vi "convertDataNiDAQmx.vi"(8 "error in (no error)":errorcluster, 10 "Data":T1={"Timestamps ms"=[0.0, 0.005, 0.009, 0.012], "Bitmap"=[[TRUE, FALSE, FALSE, FALSE, FALSE, FALSE, FALSE, FALSE, FALSE, TRUE, TRUE, FALSE, FALSE, FALSE, FALSE, FALSE], [FALSE, FALSE, FALSE, FALSE, FALSE, FALSE, FALSE, FALSE, FALSE, FALSE, FALSE, FALSE, FALSE, FALSE, FALSE, TRUE], [FALSE, FALSE, FALSE, FALSE, TRUE, FALSE, FALSE, FALSE, FALSE, FALSE, FALSE, FALSE, FALSE, FALSE, FALSE, FALSE]]} {"Timestamps ms" format="%.3f"}, 11 "niDAQmxDO in":refnum<class "niDAQmxDO.lvclass">) -> (0 "error out":errorcluster, 3 "niDAQmxDO out":refnum<class "niDAQmxDO.lvclass">)   [LabVIEW 2009, in "Hardware.lvlib" / "Channels.lvlib" / "niDAQmxDO.lvclass"]
uses:
  niDAQmxDO.lvclass
  <vilib>/Waveform/DWDTOps.llb/DWDT Append Digital Samples.vi
  <vilib>/Waveform/DWDTOps.llb/Digital Pattern Generator (Single Value).vi
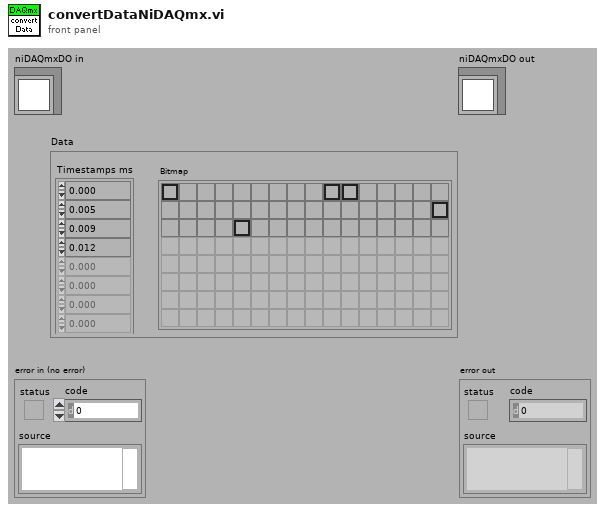
[diagram p1: front panel]
types:
  T1 = cluster{"Timestamps ms":dbl[], "Bitmap":bool[][]}
  T2 = cluster{"Master Clock source":string, "Master Clock rate":dbl, "Start trigger line":string, "Scan rate":dbl, "Stop trigger line":string, "Sample Number":dbl}
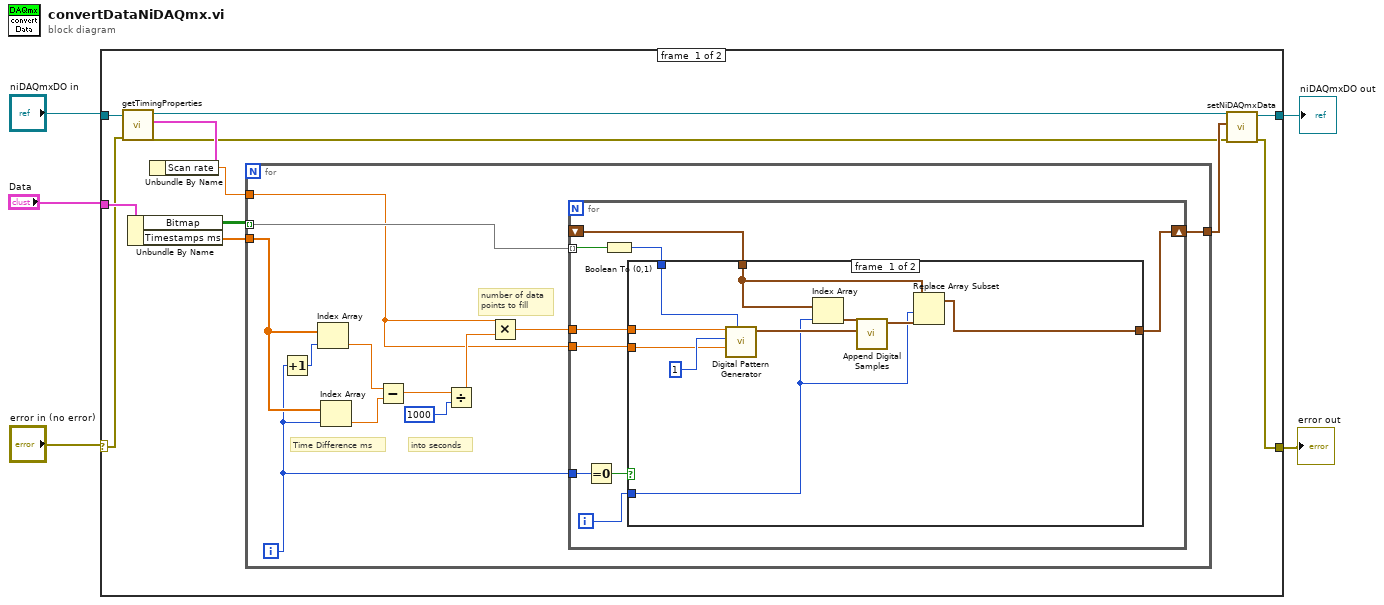
[diagram p0: block diagram]
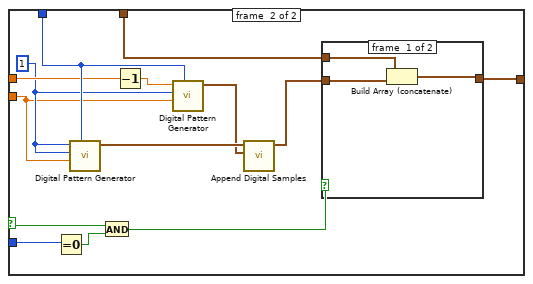
[diagram p2: hidden frame]
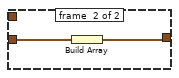
[diagram p3: hidden frame]
diagram:
  n1 = case shown="No Error" "error in (no error)" {
    selector: "error in (no error)" -> [w14 w69]
    tunnel: [w6 w69] -> w4
    tunnel: [w10 w68] -> w2
    tunnel: "niDAQmxDO in" -> [w13 w68]
    tunnel: "Data" -> [w17 _]
    frame #0 {
      n2 = call-dynamic "getTimingProperties.vi"("error in (no error)"=w14, "DigitalOutput.lvclass in"=w13) -> ("error out"=w7:errorcluster, "Timing"=w12:T2, "DigitalOutput.lvclass out"=w8:refnum<class "niDAQmxDO.lvclass">)  [unwired: 7 in]
      n3 = Unbundle By Name(w17) -> ("Bitmap"=w16:bool[][], "Timestamps ms"=w15:dbl[])
      n4 = Unbundle By Name(w12) -> ("Scan rate"=w11:dbl)
      n5 = for {
        tunnel: w16 -> [w22] mode=indexing
        tunnel: w15 -> [w26]
        tunnel: [w21] -> w9
        tunnel: w11 -> [w18]
        i -> [w20]
        # "into seconds"
        # "number of data\npoints to fill"
        # "Time Difference ms"
        n6 = Increment(x=w20) -> (x+1=w28:i32)
        n7 = Index Array(array=w26, index=w28) -> (element=w29:dbl)
        n8 = Index Array(array=w26, index=w20) -> (element=w27:dbl)
        n9 = Subtract(x=w29, y=w27) -> (x-y=w24:dbl)
        n10 = Divide(x=w24, y=1000) -> (x/y=w25:dbl)
        n11 = Multiply(x=w18, y=w25) -> (x*y=w19:dbl)
        n12 = for {
          tunnel: w19 -> [w38]
          tunnel: w22 -> [w37] mode=indexing
          shift-right: [w32] -> w21
          shift-left: _ -> [w31]
          tunnel: w20 -> [w35]
          tunnel: w18 -> [w30]
          i -> [w33]
          n13 = Equal To 0?(x=w35) -> (x = 0?=w34:bool)
          n14 = Boolean To (0,1)(Boolean=w37) -> (0, 1=w36:i16)
          n15 = case shown="True" w34 {
            selector: w34 -> [_ w60]
            tunnel: w38 -> [w47 w55]
            tunnel: w36 -> [w46 w56]
            tunnel: [w40 w62] -> w32
            tunnel: w33 -> [w41 w58]
            tunnel: w31 -> [w43 w57]
            tunnel: w30 -> [w39 w49]
            frame #0 {
              n16 = call-poly <vilib>:"Digital Pattern Generator.vi"("value"=w46, "sample rate"=w39, "number of signals"=1, "number of samples"=w47) -> ("digital waveform"=w44:digitalwaveform)  [unwired: 6 in, 1 out]
              n17 = Index Array(array=w43, index=w41) -> (element=w45:digitalwaveform)
              n18 = call-poly <vilib>:"Append Digital Samples.vi"("digital waveform B"=w44, "digital waveform A"=w45) -> ("digital waveform out"=w42:digitalwaveform)  [unwired: 8 in, 1 out]
              n19 = Replace Array Subset(array=w43, new element=w42, index=w41) -> (w40:digitalwaveform[])
            }
            frame #1 {
              w54 = 1
              n20 = Equal To 0?(x=w58) -> (x = 0?=w59:bool)
              n21 = call-poly <vilib>:"Digital Pattern Generator.vi"("value"=w56, "sample rate"=w49, "number of signals"=w54, "number of samples"=w54) -> ("digital waveform"=w53:digitalwaveform)  [unwired: 6 in, 1 out]
              n22 = And(x=w60, y=w59) -> (x .and. y?=w61:bool)
              n23 = Decrement(x=w55) -> (x-1=w50:dbl)
              n24 = call-poly <vilib>:"Digital Pattern Generator.vi"("value"=w56, "sample rate"=w49, "number of signals"=w54, "number of samples"=w50) -> ("digital waveform"=w52:digitalwaveform)  [unwired: 6 in, 1 out]
              n25 = call-poly <vilib>:"Append Digital Samples.vi"("digital waveform B"=w52, "digital waveform A"=w53) -> ("digital waveform out"=w51:digitalwaveform)  [unwired: 8 in, 1 out]
              n26 = case shown="False" w61 {
                tunnel: [w64 w67] -> w62
                tunnel: w57 -> [w65 _]
                tunnel: w51 -> [w63 w66]
                frame #0 {
                  n27 = Build Array (concatenate)(w65, w63) -> (w64:digitalwaveform[])
                }
                frame #1 {
                  n28 = Build Array(w66) -> (w67:digitalwaveform[])
                }
              }
            }
          }
        }
      }
      n29 = call "setNiDAQmxData.vi"("error in (no error)"=w7, "NIDAQmx data format"=w9, "niDAQmxDO.lvclass in"=w8) -> ("error out"=w6:errorcluster, "niDAQmxDO.lvclass out"=w10:refnum<class "niDAQmxDO.lvclass">)  [unwired: 7 in]
    }
    frame #1 {
    }
  }
  "error out" <- w4
  "niDAQmxDO out" <- w2
